vi "波形图.vi"() -> ()   [LabVIEW 2014]
uses:
  <vilib>/Native 3D Graph/xcontrol/3DPC_SurfacePlot.xctl
panel:
  out "3D Graph 2":refnum<class "Base Datatype.lvclass">[](xcontrol) caption="三维图形"
  out "3D Graph":refnum<class "Base Datatype.lvclass">[](xcontrol) caption="三维图形"
  in  "数字数据":digitaldata
  out "数字波形图 2":digitalwaveform(graph)
  out "数字波形图":digitaldata(graph)
  out "XY Graph":cluster{"Y":dbl[], "Y":dbl[]}[](graph) caption="XY图"
  in  "相移":dbl(knob) scale=0.0..10.0
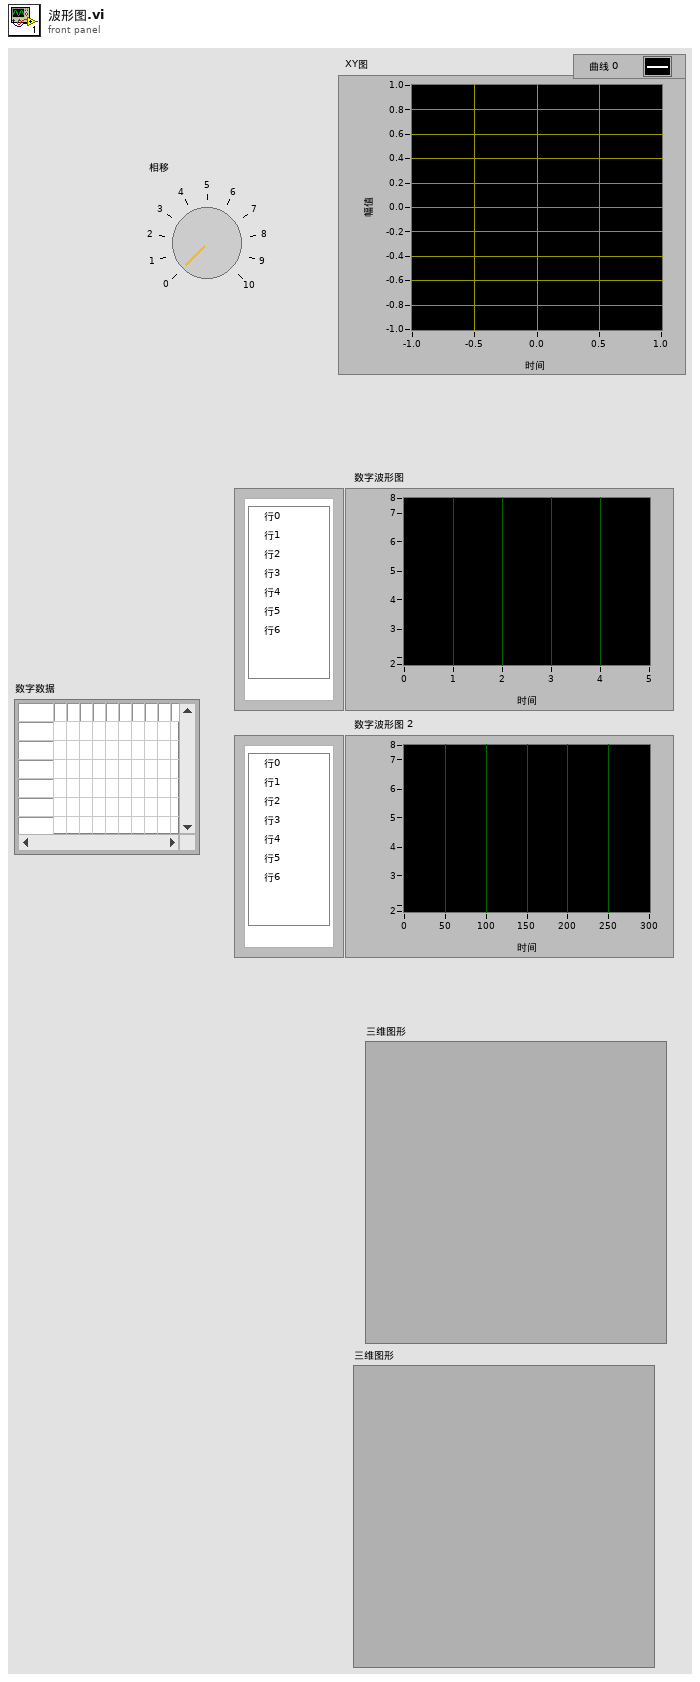
[diagram p1: front panel]
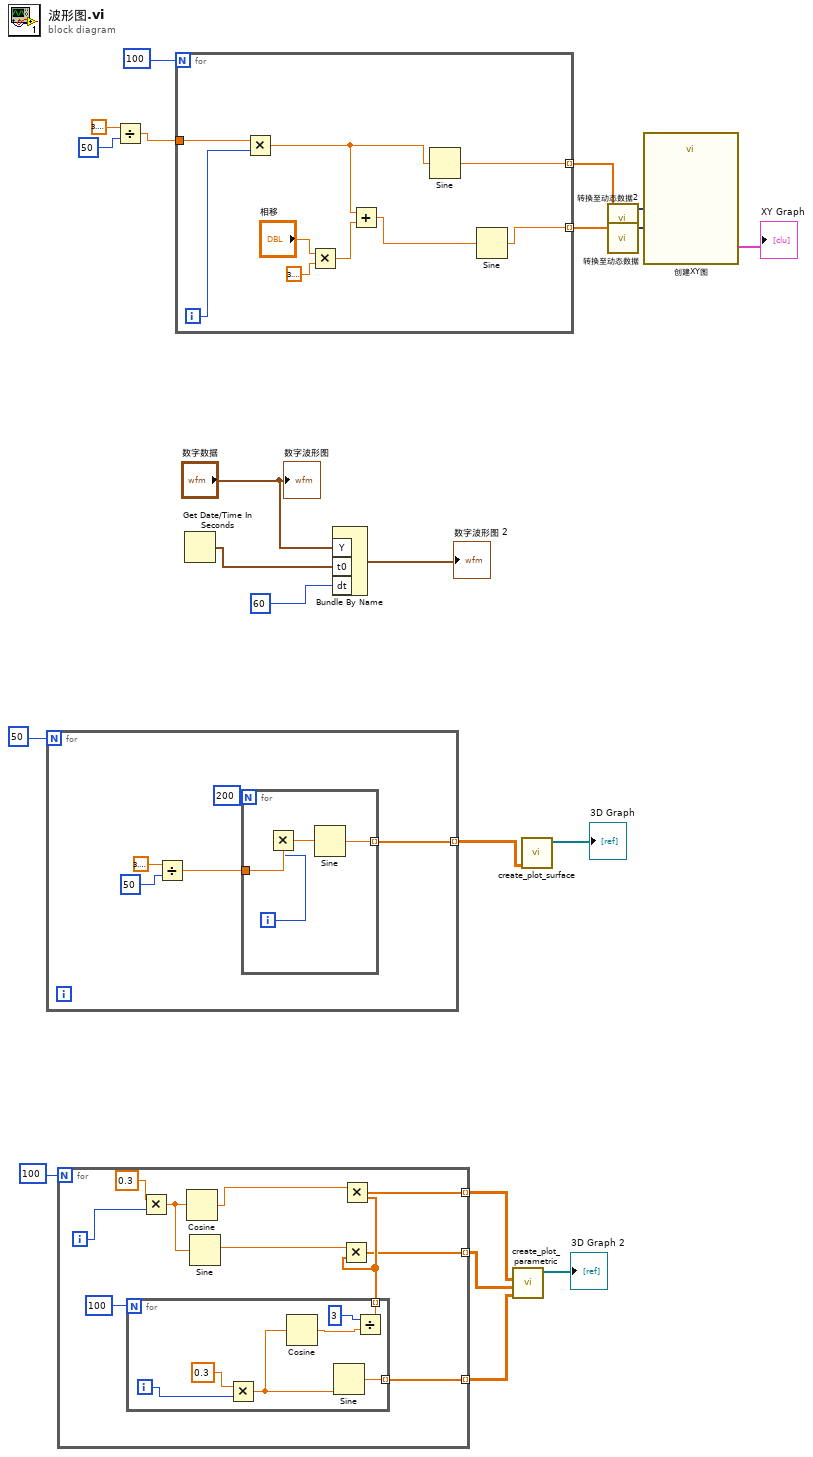
[diagram p0: block diagram]
diagram:
  n1 = for {
    N: 50 -> [_]
    tunnel: [w26] -> w6 mode=indexing
    n2 = Divide(x=3.141592653589793, y=50) -> (x/y=w22:dbl)
    n3 = for {
      N: 200 -> [_]
      tunnel: [w30] -> w26 mode=indexing
      tunnel: w22 -> [w29]
      i -> [w28]
      n4 = Multiply(x=w29, y=w28) -> (x*y=w27:dbl)
      n5 = Sine(x=w27) -> (sin(x)=w30:dbl)
    }
  }
  n6 = for {
    N: 100 -> [_]
    tunnel: [w33] -> w3 mode=indexing
    tunnel: [w32] -> w2 mode=indexing
    tunnel: [w31] -> w1 mode=indexing
    i -> [w40]
    n7 = for {
      N: 100 -> [_]
      tunnel: [w42] -> w35 mode=indexing
      tunnel: [w41] -> w31 mode=indexing
      i -> [w45]
      n8 = Multiply(x=0.3, y=w45) -> (x*y=w43:dbl)
      n9 = Cosine(x=w43) -> (cos(x)=w46:dbl)
      n10 = Sine(x=w43) -> (sin(x)=w41:dbl)
      n11 = Divide(x=3, y=w46) -> (x/y=w42:dbl)
    }
    n12 = Multiply(x=0.3, y=w40) -> (x*y=w37:dbl)
    n13 = Cosine(x=w37) -> (cos(x)=w36:dbl)
    n14 = Sine(x=w37) -> (sin(x)=w34:dbl)
    n15 = Multiply(x=w34, y=w35) -> (x*y=w32:dbl[])
    n16 = Multiply(x=w36, y=w35) -> (x*y=w33:dbl[])
  }
  n17 = Divide(x=3.141592653589793, y=50) -> (x/y=w17:dbl)
  n18 = for {
    N: 100 -> [_]
    tunnel: w17 -> [w56]
    tunnel: [w49] -> w16 mode=indexing
    tunnel: [w48] -> w14 mode=indexing
    i -> [w55]
    n19 = Multiply(x=w56, y=w55) -> (x*y=w51:dbl)
    n20 = Multiply(x="相移", y=3.141592653589793) -> (x*y=w52:dbl)
    n21 = Add(x=w51, y=w52) -> (x+y=w50:dbl)
    n22 = Sine(x=w51) -> (sin(x)=w48:dbl)
    n23 = Sine(x=w50) -> (sin(x)=w49:dbl)
  }
  n24 = Get Date/Time In Seconds() -> (seconds since 1Jan1904=w11:timestamp)
  n25 = Bundle By Name ("创建波形")("Y"="数字数据", "t0"=w11, "dt"=60) -> (→"数字波形图 2":digitalwaveform)  [unwired: 1 in]
  n26 = call <vilib>:"create_plot_parametric.vi"("z matrix"=w1, "y matrix"=w2, "x matrix"=w3) -> ("plots out"=→"3D Graph 2":refnum<class "Base Datatype.lvclass">[])  [unwired: 2 in, 6 out]
  n27 = call <vilib>:"create_plot_surface.vi"("z matrix"=w6) -> ("plots out"=→"3D Graph":refnum<class "Base Datatype.lvclass">[])  [unwired: 4 in, 6 out]
  n28 = call "转换至动态数据2"("Array"=w14) -> ("Dynamic Data Type"=w13:dynamicdata)  [unwired: 3 in]
  n29 = call "转换至动态数据"("Array"=w16) -> ("Dynamic Data Type"=w15:dynamicdata)  [unwired: 3 in]
  n30 = call "创建XY图"("Y Input"=w15, "X Input"=w13) -> ("XY Graph"=→"XY Graph":cluster{"X":dbl[], "Y":dbl[]}[])  [unwired: 8 in, 1 out]
  "数字波形图" <- "数字数据"
